vi "ACC_LabVIEW_Call.vi"(0 "DeviceReferenceIn":cluster{"ID":u32}, 2 "Propname":string, 3 "Acc_Para_In":T1[](array[typedef]), 5 "error in (no error)":errorcluster, 7 "Error strings buffer size (Byte)":u32=500, 8 "VirtAcc":i32) -> (14 "DeviceReferenceOut":cluster{"ID":u32}, 19 "error out":errorcluster)   [LabVIEW 2014, in "ACC_LabVIEW.lvlib"]
doc: "Perform a call inside the GSI - accelerator control system."
uses:
  ACC_LabVIEW.lvlib
  ACC_LabVIEW_Container.ctl
  ACC_LabVIEW_DataTypes.ctl
  lib/ACC_Interface_Wrapper.dll
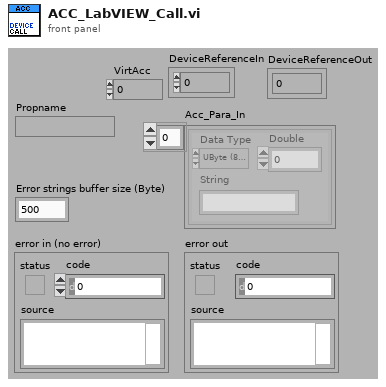
[diagram p1: front panel]
types:
  T1 = typedef "ACC_LabVIEW.lvlib/ACC_LabVIEW_Container.ctl" = cluster{"Data Type":T2, "String":string, "Double":dbl}
  T2 = typedef "ACC_LabVIEW.lvlib/ACC_LabVIEW_DataTypes.ctl" = enum16{"SByte (8Bit Int signed)", "UByte (8Bit int unsigned)", "SWord (16Bit Int signed)", "UWord (16Bit Int unsigned)", "SLong (32Bit Int signed)", "ULong (32Bit Int unsigned)", "Float32 (float)", "Float64 (double)", "String"}
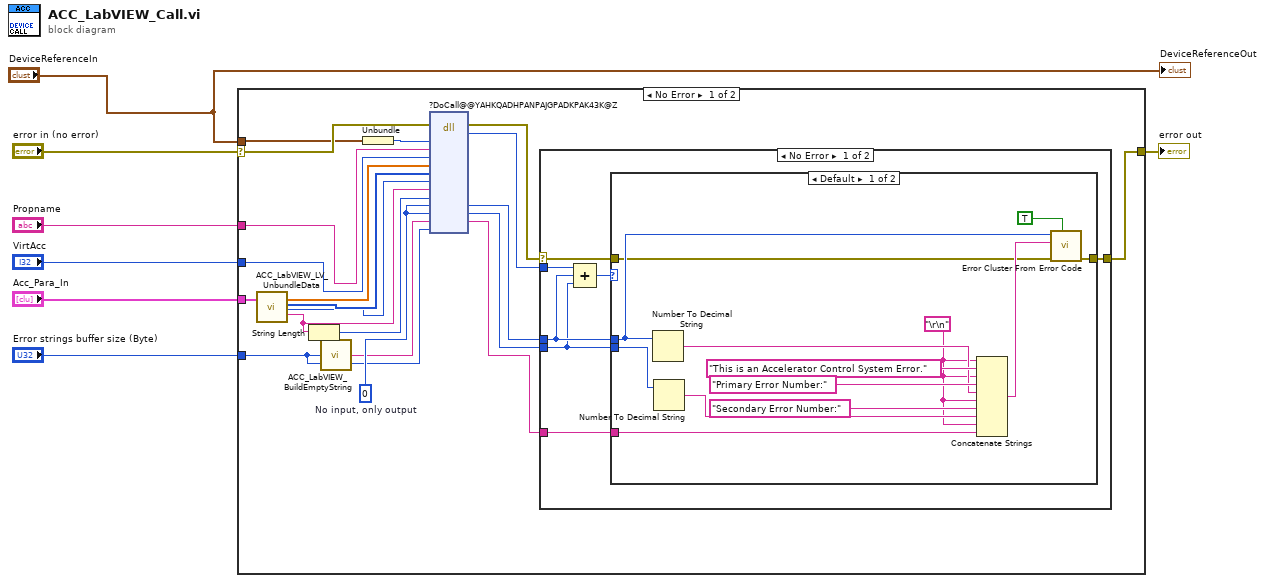
[diagram p0: block diagram]
diagram:
  n1 = case shown="No Error" "error in (no error)" {
    selector: "error in (no error)" -> [w25 w50]
    tunnel: "Propname" -> [w24 _]
    tunnel: "VirtAcc" -> [w23 _]
    tunnel: [w27 w50] -> w5
    tunnel: "Error strings buffer size (Byte)" -> [w15 _]
    tunnel: "Acc_Para_In" -> [w26 _]
    tunnel: "DeviceReferenceIn" -> [w9 _]
    frame No Error {
      w17 = u32 0  # No input, only output
      n2 = call "ACC_LabVIEW_LV_UnbundleData.vi"("Acc_Data_In"=w26) -> ("LV_double_array"=w22:dbl[], "LV_types"=w21:i32[], "Length"=w20:i32, "Data-String"=w19:string)  [unwired: 15 in]
      n3 = String Length(string=w19) -> (length=w18:i32)
      n4 = call "ACC_LabVIEW_BuildEmptyString.vi"("Length"=w15) -> ("String"=w16:string)
      n5 = Unbundle(w9) -> ("ID"=w8:u32)
      n6 = dll-call lib="D:/Git/CS-framework/CSinstr.lib/ACC_LabVIEW_Interface/lib/ACC_Interface_Wrapper.dll" fn="?DoCall@@YAHKQADHPANPAJGPADKPAK43K@Z"(error in=w25, "DeviceHandle"=w8, "LV_propname"=w24, "LV_VirtAcc"=w23, "LV_para"=w22, "LV_para_types"=w21, "LV_para_Size"=w20, "LV_para_string"=w19, "LV_para_string_Size"=w18, "ErrPrimStat"=w17, "ErrSecStat"=w17, "ErrorMSG"=w16, "ErrorMSG_Size"=w15) -> (error out=w14:errorcluster, "return type"=w13:i32, "ErrPrimStat"=w12:u32, "ErrSecStat"=w11:u32, "ErrorMSG"=w10:string)  [unwired: 11 in, 1 out]
      n7 = case shown="No Error" w14 {
        selector: w14 -> [w32 w49]
        tunnel: w13 -> [w34 _]
        tunnel: [w31 w49] -> w27
        tunnel: w12 -> [w29 _]
        tunnel: w11 -> [w28 _]
        tunnel: w10 -> [w30 _]
        frame No Error {
          n8 = Compound Arithmetic op=ADD(w34, w29, w28) -> (w33:u32)
          n9 = case shown="Default" w33 {
            tunnel: w32 -> [w37 w48]
            tunnel: [w36 w48] -> w31
            tunnel: w29 -> [w38 _]
            tunnel: w28 -> [w42 _]
            tunnel: w30 -> [w40 _]
            frame Default {
              w41 = "\r\n"
              n10 = Number To Decimal String(number=w38) -> (decimal integer string=w45:string)  [unwired: 1 in]
              n11 = Number To Decimal String(number=w42) -> (decimal integer string=w43:string)  [unwired: 1 in]
              n12 = Concatenate Strings(w41, "This is an Accelerator Control System Error.", w41, "Primary Error Number:", w45, w41, "Secondary Error Number:", w43, w41, w40) -> (w39:string)
              n13 = call <vilib>:"Error Cluster From Error Code.vi"("show call chain? (False)"=TRUE, "error in (no error)"=w37, "error message (\"\")"=w39, "error code (0)"=w38) -> ("error out"=w36:errorcluster)  [unwired: 5 in]
            }
            frame 0 {
              # "no error"
            }
          }
        }
        frame Error {
        }
      }
    }
    frame Error {
    }
  }
  "error out" <- w5
  "DeviceReferenceOut" <- "DeviceReferenceIn"
